vi "experiment control.vi"() -> ()   [LabVIEW 2012] (continued)
                  tunnel: w3124 -> [w3135]
                  stop <- w3140 stop-if-true
                  n1342 = Multiply(x=w3136, y=0.001) -> (x*y=w3144:dbl)
                  n1343 = call-poly <vilib>:"DAQmx Create Virtual Channel.vi"("maximum value"=10.0, "minimum value"=0.0, "physical channels"=w3146, "error in"=w3135) -> ("task out"=w3155:refnum<k21>, "error out"=w3154:errorcluster)  [unwired: 10 in]
                  n1344 = Add(x=w3139, y=w3144) -> (x+y=w3143:dbl)
                  n1345 = Max & Min(x=w3139, y=w3134) -> (max(x,y)=w3142:dbl, min(x,y)=w3141:dbl)
                  n1346 = In Range and Coerce(upper limit=w3142, x=w3143, lower limit=w3141) -> (coerced(x)=w3137:dbl)  [unwired: 1 out]
                  n1347 = call-poly <vilib>:"DAQmx Write.vi"("task/channels in"=w3155, "data"=w3137, "error in"=w3154) -> ("task out"=w3151:refnum<k21>, "error out"=w3156:errorcluster)  [unwired: 10 in, 1 out]
                  n1348 = Equal?(x=w3137, y=w3134) -> (x = y?=w3140:bool)
                  n1349 = call <vilib>:"DAQmx Start Task.vi"("task/channels in"=w3151, "error in"=w3156) -> ("task out"=w3150:refnum<k21>, "error out"=w3149:errorcluster)  [unwired: 12 in]
                  n1350 = call <vilib>:"DAQmx Clear Task.vi"("task in"=w3150, "error in"=w3149) -> ("error out"=w3148:errorcluster)  [unwired: 13 in]
                  n1351 = call "wait.vi"("error in (no error)"=w3148, "ms to wait"=u32 5) -> ("error out (no error)"=w3147:errorcluster)  [unwired: 7 in]
                }
              }
              frame "Stella" {
                n1352 = disable-structure shown="Disabled" {
                  disable-tunnel: w3158 -> [w3160 w3190]
                  disable-tunnel: [w3159 w3190] -> w3157
                  frame Disabled {
                    n1353 = flat-sequence {
                      tunnel: [w3165] -> w3162
                      tunnel: [w3164] -> w3161
                      tunnel: w3160 -> [w3163]
                      tunnel: w3162 -> [w3172]
                      tunnel: w3161 -> [w3170]
                      tunnel: [w3169] -> w3159
                      frame #0 {
                        n1354 = local read "Stella"() -> (w3168:T20)
                        n1355 = Unbundle By Name(w3168) -> ("scan start"=w3166:dbl)
                        n1356 = Bundle By Name(cluster=w3168, "setpoint"=w3166, "progress"=u8 0 ("number")) -> (w3165:T20)
                        n1357 = shared-variable "My Computer\\shared variables.lvlib\\lisa setpoint"(w3166, error in=w3163) -> (error out=w3164:errorcluster)
                        n1358 = local write "Stella"(w3165) -> ()
                      }
                      frame #1 {
                        n1359 = Tick Count (ms)() -> (millisecond timer value=w3171:u32)
                        n1360 = while {
                          tunnel: w3172 -> [w3189]
                          tunnel: w3171 -> [w3184]
                          shift-right: [w3173] -> w3169
                          shift-left: w3170 -> [w3174]
                          stop <- w3179 stop-if-true
                          n1361 = shared-variable "My Computer\\shared variables.lvlib\\lisa wavelength"(error in=w3174) -> (w3175:dbl, error out=w3173:errorcluster)
                          n1362 = Unbundle By Name(w3189) -> ("setpoint"=w3178:dbl, "lock tolerance"=w3186:dbl)
                          n1363 = Subtract(x=w3175, y=w3178) -> (x-y=w3188:dbl)
                          n1364 = Absolute Value(x=w3188) -> (abs(x)=w3187:dbl)
                          n1365 = Less?(x=w3187, y=w3186) -> (x < y?=w3180:bool)
                          n1366 = local read "Stella"() -> (w3176:T20)
                          n1367 = Bundle By Name(cluster=w3176, "wavelength"=w3175) -> (w3177:T20)
                          n1368 = Tick Count (ms)() -> (millisecond timer value=w3185:u32)
                          n1369 = Subtract(x=w3185, y=w3184) -> (x-y=w3183:u32)
                          n1370 = Greater?(x=w3183, y=u32 10000) -> (0:w3181:bool)
                          n1371 = local write "Stella"(w3177) -> ()
                          n1372 = Or(x=w3180, y=w3181) -> (x .or. y?=w3179:bool)
                        }
                      }
                    }
                  }
                  frame Enabled {
                  }
                }
              }
              frame "Jessica" {
                n1373 = disable-structure shown="Enabled" {
                  disable-tunnel: w3192 -> [w3194 w3224]
                  disable-tunnel: [w3193 w3224] -> w3191
                  frame Disabled {
                    n1374 = flat-sequence {
                      tunnel: [w3199] -> w3196
                      tunnel: [w3198] -> w3195
                      tunnel: w3194 -> [w3197]
                      tunnel: w3196 -> [w3206]
                      tunnel: w3195 -> [w3204]
                      tunnel: [w3203] -> w3193
                      frame #0 {
                        n1375 = local read "Jessica"() -> (w3202:T17)
                        n1376 = Unbundle By Name(w3202) -> ("scan start"=w3200:dbl)
                        n1377 = Bundle By Name(cluster=w3202, "setpoint"=w3200, "progress"=u8 0 ("number")) -> (w3199:T17)
                        n1378 = shared-variable "My Computer\\shared variables.lvlib\\jessica setpoint"(w3200, error in=w3197) -> (error out=w3198:errorcluster)
                        n1379 = local write "Jessica"(w3199) -> ()
                      }
                      frame #1 {
                        n1380 = Tick Count (ms)() -> (millisecond timer value=w3205:u32)
                        n1381 = while {
                          tunnel: w3206 -> [w3223]
                          tunnel: w3205 -> [w3218]
                          shift-right: [w3207] -> w3203
                          shift-left: w3204 -> [w3208]
                          stop <- w3213 stop-if-true
                          n1382 = shared-variable "My Computer\\shared variables.lvlib\\jessica wavelength"(error in=w3208) -> (w3209:dbl, error out=w3207:errorcluster)
                          n1383 = Unbundle By Name(w3223) -> ("setpoint"=w3212:dbl, "lock tolerance"=w3220:dbl)
                          n1384 = Subtract(x=w3209, y=w3212) -> (x-y=w3222:dbl)
                          n1385 = Absolute Value(x=w3222) -> (abs(x)=w3221:dbl)
                          n1386 = Less?(x=w3221, y=w3220) -> (x < y?=w3214:bool)
                          n1387 = local read "Jessica"() -> (w3210:T17)
                          n1388 = Bundle By Name(cluster=w3210, "wavelength"=w3209) -> (w3211:T17)
                          n1389 = Tick Count (ms)() -> (millisecond timer value=w3219:u32)
                          n1390 = Subtract(x=w3219, y=w3218) -> (x-y=w3217:u32)
                          n1391 = Greater?(x=w3217, y=u32 10000) -> (0:w3215:bool)
                          n1392 = local write "Jessica"(w3211) -> ()
                          n1393 = Or(x=w3214, y=w3215) -> (x .or. y?=w3213:bool)
                        }
                      }
                    }
                  }
                  frame Enabled {
                  }
                }
              }
              frame "Bertha" {
                n1394 = local read "Bertha"() -> (w3229:T22)
                n1395 = Unbundle By Name(w3229) -> ("scan start"=w3227:dbl)
                n1396 = Bundle By Name(cluster=w3229, "setpoint"=w3227, "progress"=u8 0 ("number")) -> (w3228:T22)
                n1397 = local write "Bertha"(w3228) -> ()
              }
              frame "Cora" {
                n1398 = local read "Cora"() -> (w3234:T21)
                n1399 = Unbundle By Name(w3234) -> ("scan start"=w3232:dbl)
                n1400 = Bundle By Name(cluster=w3234, "setpoint"=w3232, "progress"=u8 0 ("number")) -> (w3233:T21)
                n1401 = local write "Cora"(w3233) -> ()
              }
            }
          }
          frame "Laser: Read Wavelength" {
            n1402 = case shown="\"Stella\"" w3238 {
              tunnel: [w3240 w3242 w3270 w3289 w3308 w3337] -> w3236
              tunnel: w3237 -> [w3240 w3241 w3272 w3293 w3307 w3338]
              frame Default {
              }
              frame "Jessica" {
                n1403 = disable-structure shown="Enabled" {
                  disable-tunnel: [w3249 w3264] -> w3242
                  disable-tunnel: w3241 -> [w3253 w3264]
                  frame Enabled {
                    n1404 = disable-structure shown="Enabled" {
                      disable-tunnel: w3253 -> [w3258 w3261]
                      disable-tunnel: [w3257 w3259] -> w3250
                      disable-tunnel: [w3256 w3260] -> w3249
                      frame Disabled {
                        n1405 = shared-variable "My Computer\\shared variables.lvlib\\luna_wavelength"(error in=w3258) -> (w3257:dbl, error out=w3256:errorcluster)
                      }
                      frame Enabled {
                        n1406 = call "read_cw.vi"("error in"=w3261, "cw_laser"="cw3") -> ("error out"=w3260:errorcluster, "slot"=w3262:T101)  [unwired: 8 in]
                        n1407 = Unbundle By Name(w3262) -> ("wavelength"=w3259:dbl)
                      }
                    }
                    n1408 = local read "Jessica"() -> (w3254:T17)
                    n1409 = Unbundle By Name(w3254) -> ("wavelength"=w3251:dbl, "setpoint"=w3245:dbl, "lock tolerance"=w3243:dbl)
                    n1410 = Less Or Equal To 0?(x=w3250) -> (x <= 0?=w3252:bool)
                    n1411 = Select(t=w3251, s=w3252, f=w3250) -> (s? t:f=w3244:dbl)
                    n1412 = Subtract(x=w3245, y=w3244) -> (x-y=w3248:dbl)
                    n1413 = Absolute Value(x=w3248) -> (abs(x)=w3247:dbl)
                    n1414 = Less?(x=w3247, y=w3243) -> (x < y?=w3246:bool)
                    n1415 = Bundle By Name(cluster=w3254, "locked"=w3246, "wavelength"=w3244) -> (w3255:T17)
                    n1416 = local write "Jessica"(w3255) -> ()
                  }
                  frame Disabled {
                  }
                }
              }
              frame "Toptica" {
                n1417 = local read "Toptica"() -> (w3276:T19)
                n1418 = disable-structure shown="Enabled" {
                  disable-tunnel: [w3280 w3281] -> w3273
                  disable-tunnel: w3272 -> [w3279 w3284]
                  disable-tunnel: [w3278 w3283] -> w3266
                  frame Disabled {
                    n1419 = shared-variable "My Computer\\shared variables.lvlib\\toptica_wavelength"(error in=w3279) -> (w3280:dbl, error out=w3278:errorcluster)
                  }
                  frame Enabled {
                    n1420 = call "read_cw.vi"("error in"=w3284, "cw_laser"="cw1") -> ("error out"=w3283:errorcluster, "slot"=w3282:T101)  [unwired: 8 in]
                    n1421 = Unbundle By Name(w3282) -> ("wavelength"=w3281:dbl)
                  }
                }
                n1422 = Unbundle By Name(w3276) -> ("wavelength"=w3274:dbl)
                n1423 = Less Or Equal To 0?(x=w3273) -> (x <= 0?=w3275:bool)
                n1424 = Select(t=w3274, s=w3275, f=w3273) -> (s? t:f=w3271:dbl)
                n1425 = local read "toptica:task:skip"() -> (w3265:refnum<k21>)
                n1426 = call-poly <vilib>:"DAQmx Read.vi"("task/channels in"=w3265, "error in"=w3266) -> ("data"=w3268:dbl, "error out"=w3270:errorcluster)  [unwired: 11 in, 1 out]
                n1427 = Less?(x=w3268, y=1.8) -> (x < y?=w3269:bool)
                n1428 = Bundle By Name(cluster=w3276, "locked"=w3269, "wavelength"=w3271) -> (w3277:T19)
                n1429 = local write "Toptica"(w3277) -> ()
              }
              frame "Stella" {
                n1430 = disable-structure shown="Enabled" {
                  disable-tunnel: [w3301 w3303] -> w3294
                  disable-tunnel: w3293 -> [w3300 w3302]
                  disable-tunnel: [w3299 w3304] -> w3287
                  frame Disabled {
                    n1431 = shared-variable "My Computer\\shared variables.lvlib\\stella_wavelength"(error in=w3300) -> (w3301:dbl, error out=w3299:errorcluster)
                  }
                  frame Enabled {
                    n1432 = call "read_cw.vi"("error in"=w3302, "cw_laser"="cw0") -> ("error out"=w3304:errorcluster, "slot"=w3305:T101)  [unwired: 8 in]
                    n1433 = Unbundle By Name(w3305) -> ("wavelength"=w3303:dbl)
                  }
                }
                n1434 = local read "Stella"() -> (w3297:T20)
                n1435 = Unbundle By Name(w3297) -> ("wavelength"=w3295:dbl)
                n1436 = Less Or Equal To 0?(x=w3294) -> (x <= 0?=w3296:bool)
                n1437 = Select(t=w3295, s=w3296, f=w3294) -> (s? t:f=w3292:dbl)
                n1438 = local read "stella:task:skip"() -> (w3286:refnum<k21>)
                n1439 = call-poly <vilib>:"DAQmx Read.vi"("task/channels in"=w3286, "error in"=w3287) -> ("data"=w3291:dbl, "error out"=w3289:errorcluster)  [unwired: 11 in, 1 out]
                n1440 = Less?(x=w3291, y=1.8) -> (x < y?=w3288:bool)
                n1441 = Bundle By Name(cluster=w3297, "locked"=w3288, "wavelength"=w3292) -> (w3298:T20)
                n1442 = local write "Stella"(w3298) -> ()
              }
              frame "Cora" {
                n1443 = disable-structure shown="Enabled" {
                  disable-tunnel: [w3309 w3330] -> w3308
                  disable-tunnel: w3307 -> [w3312 w3330]
                  frame Enabled {
                    n1444 = disable-structure shown="Enabled" {
                      disable-tunnel: [w3319 w3320] -> w3313
                      disable-tunnel: w3312 -> [w3318 w3323]
                      disable-tunnel: [w3317 w3322] -> w3309
                      frame Disabled {
                        n1445 = shared-variable "My Computer\\shared variables.lvlib\\cora_wavelength"(error in=w3318) -> (w3319:dbl, error out=w3317:errorcluster)
                      }
                      frame Enabled {
                        n1446 = disable-structure shown="Enabled" {
                          disable-tunnel: "pulse1" ("cw_laser") -> [w3328 _]
                          disable-tunnel: w3323 -> [w3327 w3329]
                          disable-tunnel: [w3326 w3329] -> w3322
                          disable-tunnel: [w3325 _] -> w3321
                          frame Disabled {
                            n1447 = call "read_pulsed.vi"("error in"=w3327, "pulsed_laser"=w3328) -> ("error out"=w3326:errorcluster, "slot"=w3325:T102)  [unwired: 8 in]
                          }
                          frame Enabled {
                          }
                        }
                        n1448 = Unbundle By Name(w3321) -> ("wavelength"=w3320:dbl)
                      }
                    }
                    n1449 = local read "Cora"() -> (w3315:T21)
                    n1450 = Unbundle By Name(w3315) -> ("wavelength"=w3310:dbl)
                    n1451 = Less Or Equal To 0?(x=w3313) -> (x <= 0?=w3314:bool)
                    n1452 = Select(t=w3310, s=w3314, f=w3313) -> (s? t:f=w3311:dbl)
                    n1453 = Bundle By Name(cluster=w3315, "wavelength"=w3311) -> (w3316:T21)
                    n1454 = local write "Cora"(w3316) -> ()
                  }
                  frame Disabled {
                  }
                }
              }
              frame "Bertha" {
                n1455 = local read "Bertha"() -> (w3334:T22)
                n1456 = Unbundle By Name(w3334) -> ("wavelength"=w3333:dbl)
                n1457 = disable-structure shown="Enabled" {
                  disable-tunnel: [w3341 w3342] -> w3331
                  disable-tunnel: w3338 -> [w3340 w3345]
                  disable-tunnel: [w3339 w3344] -> w3337
                  frame Disabled {
                    n1458 = shared-variable "My Computer\\shared variables.lvlib\\cora_wavelength"(error in=w3340) -> (w3341:dbl, error out=w3339:errorcluster)
                  }
                  frame Enabled {
                    n1459 = disable-structure shown="Disabled" {
                      disable-tunnel: "pulse1" ("cw_laser") -> [w3350 _]
                      disable-tunnel: w3345 -> [w3349 w3351]
                      disable-tunnel: [w3348 w3351] -> w3344
                      disable-tunnel: [w3347 _] -> w3343
                      frame Disabled {
                        n1460 = call "read_pulsed.vi"("error in"=w3349, "pulsed_laser"=w3350) -> ("error out"=w3348:errorcluster, "slot"=w3347:T102)  [unwired: 8 in]
                      }
                      frame Enabled {
                      }
                    }
                    n1461 = Unbundle By Name(w3343) -> ("wavelength"=w3342:dbl)
                  }
                }
                n1462 = Less Or Equal To 0?(x=w3331) -> (x <= 0?=w3336:bool)
                n1463 = Select(t=w3333, s=w3336, f=w3331) -> (s? t:f=w3332:dbl)
                n1464 = Bundle By Name(cluster=w3334, "wavelength"=w3332) -> (w3335:T22)
                n1465 = local write "Bertha"(w3335) -> ()
              }
            }
          }
          frame "Laser: Initialize DAC" {
            n1466 = local read "Toptica"() -> (w3359:T19)
            n1467 = local read "Stella"() -> (w3358:T20)
            n1468 = Unbundle By Name(w3359) -> ("AI Channel"=w3360:tag)
            n1469 = Unbundle By Name(w3358) -> ("AI Channel"=w3357:tag)
            n1470 = call-poly <vilib>:"DAQmx Create Virtual Channel.vi"("physical channels"=w3360, "error in"=w3354) -> ("task out"=→"toptica:task:skip":refnum<k21>, "error out"=w3356:errorcluster)  [unwired: 12 in]
            n1471 = call-poly <vilib>:"DAQmx Create Virtual Channel.vi"("physical channels"=w3357, "error in"=w3356) -> ("task out"=→"stella:task:skip":refnum<k21>, "error out"=w3355:errorcluster)  [unwired: 12 in]
          }
          frame "Laser: Close DAC" {
            n1472 = local read "toptica:task:skip"() -> (w3363:refnum<k21>)
            n1473 = local read "stella:task:skip"() -> (w3364:refnum<k21>)
            n1474 = call <vilib>:"DAQmx Clear Task.vi"("task in"=w3363, "error in"=w3365) -> ("error out"=w3367:errorcluster)  [unwired: 13 in]
            n1475 = call <vilib>:"DAQmx Clear Task.vi"("task in"=w3364, "error in"=w3367) -> ("error out"=w3366:errorcluster)  [unwired: 13 in]
          }
          frame "---------- Debug ----------" {
            # "Template Separator\n(You can make a copy of, or modify, this frame)"
          }
          frame "Debug: Popup" {
            # "Prints the argument to a popup dialog box. Careful! If you get stuck in a loop this can hang the program."
            n1476 = One Button Dialog(message=w3375) -> (true=w3374:bool)  [unwired: 1 in]
            n1477 = flat-sequence {
              tunnel: w3374 -> [_]
              frame #0 {
                # "This delay is added in to make it difficult for the user to create and infinite chain of popups"
                n1478 = Wait (ms)(milliseconds to wait=u32 200) -> ()  [unwired: 1 out]
              }
            }
          }
          frame "Debug: Console" {
            # "Prints the argument to the console."
            n1479 = flat-sequence {
              tunnel: w3380 -> [w3383]
              frame #0 {
                n1480 = local read "stdout"() -> (w3385:string)
                n1481 = Concatenate Strings(w3385, "\r\n", w3383) -> (w3386:string)
                n1482 = local write "stdout"(w3386) -> ()
              }
              frame #1 {
                n1483 = property on="stdout" class="Str"("Text.Scroll Position"=u32 4294967295) -> ()  [unwired: 2 in, 2 out]
              }
            }
          }
          frame "---------- Wavemaster ----------" {
            # "Template Separator\n(You can make a copy of, or modify, this frame)"
          }
          frame "Wavemeter: Initialise" {
            n1484 = local read "Wavemaster"() -> (w3397:T23)
            n1485 = Unbundle By Name(w3397) -> ("Serial Port"=w3399:refnum<visa-resource-name>)
            n1486 = Bundle By Name(cluster=T46 {"VISA resource name"="COM6", "baud rate"=9600, "data bits"=8, "parity"=0, "stop bits"=10, "flow control"=2, "termination char\n(0xA = '\\n' = LF)"=10, "timeout (ms)"=1000, "End write with termination character?"=TRUE, "End read on termination character?"=TRUE} ("Serial Settings"), "VISA resource name"=w3399) -> (w3398:T46)
            n1487 = call "Wmeter Initialize.vi"("error in"=w3402, "Serial Settings"=w3398) -> ("error out (no error)"=w3401:errorcluster, "VISA RName out"=w3396:refnum<visa-resource-name>)  [unwired: 8 in]
            n1488 = Unbundle By Name(w3401) -> ("status"=w3394:bool)
            n1489 = Not(x=w3394) -> (.not. x?=w3393:bool)
            n1490 = Bundle By Name(cluster=w3397, "VISA Name"=w3396, "Detected"=w3393) -> (w3395:T23)
            n1491 = local write "Wavemaster"(w3395) -> ()
            n1492 = Enqueue Element(queue=w3392, element="Debug: Console >> Initializing Wavemeter" ("State(s) at Back (\"\")")) -> ()  [unwired: 2 in, 3 out]
          }
          frame "Wavemeter: Start" {
            n1493 = local read "Wavemaster"() -> (w3408:T23)
            n1494 = Unbundle By Name(w3408) -> ("VISA Name"=w3407:refnum<visa-resource-name>, "Detected"=w3406:bool)
            n1495 = case shown="True" w3406 {
              tunnel: [w3413 w3420] -> w3409
              tunnel: w3410 -> [w3413 w3419]
              tunnel: w3408 -> [_ w3418]
              tunnel: w3407 -> [_ w3415]
              tunnel: ["Debug: Console >> Can't Find Wavemeter" ("State(s) at Back (\"\")") "Debug: Console >> Starting Wavemeter" ("State(s) at Back (\"\")")] -> w3405
              frame False {
              }
              frame True {
                n1496 = call "Wmeter Start.vi"("error in"=w3419, "WMeter"=w3415) -> ("error out"=w3420:errorcluster, "WMeter out"=w3417:refnum<visa-resource-name>)  [unwired: 8 in]
                n1497 = Bundle By Name(cluster=w3418, "VISA Name"=w3417) -> (w3416:T23)
                n1498 = local write "Wavemaster"(w3416) -> ()
              }
            }
            n1499 = Enqueue Element At Opposite End(queue=w3404, element=w3405) -> ()  [unwired: 2 in, 3 out]
          }
          frame "Wavemeter: Set Units" {
            n1500 = local read "Wavemaster"() -> (w3426:T23)
            n1501 = Unbundle By Name(w3426) -> ("VISA Name"=w3425:refnum<visa-resource-name>, "Units"=w3424:string, "Detected"=w3423:bool)
            n1502 = case shown="True" w3423 {
              tunnel: [w3430 w3439] -> w3427
              tunnel: w3428 -> [w3430 w3438]
              tunnel: w3426 -> [_ w3437]
              tunnel: w3425 -> [_ w3434]
              tunnel: [_ w3432] -> w3421
              tunnel: w3424 -> [_ w3431]
              frame False {
              }
              frame True {
                n1503 = call "Wmeter Units.vi"("error in"=w3438, "Combo Box"=w3431, "WMeter"=w3434) -> ("error out"=w3439:errorcluster, "WMeter out"=w3436:refnum<visa-resource-name>)  [unwired: 7 in]
                n1504 = Bundle By Name(cluster=w3437, "VISA Name"=w3436) -> (w3435:T23)
                n1505 = local write "Wavemaster"(w3435) -> ()
                n1506 = Concatenate Strings("Debug: Console >> Changing Wavemeter units to " ("State(s) at Back (\"\")"), w3431) -> (w3432:string)
              }
            }
            n1507 = Enqueue Element At Opposite End(queue=w3422, element=w3421) -> ()  [unwired: 2 in, 3 out]
          }
          frame "Wavemeter: Read" {
            n1508 = local read "Wavemaster"() -> (w3444:T23)
            n1509 = Unbundle By Name(w3444) -> ("VISA Name"=w3443:refnum<visa-resource-name>, "Wavelength"=w3442:dbl, "Detected"=w3441:bool)
            n1510 = case shown="True" w3441 {
              tunnel: [w3448 w3458] -> w3445
              tunnel: w3446 -> [w3448 w3457]
              tunnel: w3444 -> [_ w3456]
              tunnel: w3443 -> [_ w3453]
              tunnel: w3442 -> [_ w3450]
              frame False {
              }
              frame True {
                n1511 = call "Wmeter Read.vi"("error in"=w3457, "WMeter"=w3453) -> ("error out"=w3458:errorcluster, "Wavelength"=w3451:dbl, "WMeter out"=w3455:refnum<visa-resource-name>)  [unwired: 7 in]
                n1512 = Greater Than 0?(x=w3451) -> (x > 0?=w3449:bool)
                n1513 = Select(t=w3451, s=w3449, f=w3450) -> (s? t:f=w3452:dbl)
                n1514 = Bundle By Name(cluster=w3456, "VISA Name"=w3455, "Wavelength"=w3452, "Reading"=w3449) -> (w3454:T23)
                n1515 = local write "Wavemaster"(w3454) -> ()
              }
            }
          }
          frame "Wavemeter: Stop" {
            n1516 = local read "Wavemaster"() -> (w3463:T23)
            n1517 = Unbundle By Name(w3463) -> ("VISA Name"=w3462:refnum<visa-resource-name>, "Detected"=w3461:bool)
            n1518 = case shown="True" w3461 {
              tunnel: [w3467 w3474] -> w3464
              tunnel: w3465 -> [w3467 w3473]
              tunnel: w3463 -> [_ w3472]
              tunnel: w3462 -> [_ w3469]
              tunnel: [_ "Debug: Console >> Stopping Wavemeter" ("State(s) at Back (\"\")")] -> w3460
              frame False {
              }
              frame True {
                n1519 = call "Wmeter Stop.vi"("error in"=w3473, "WMeter"=w3469) -> ("error out"=w3474:errorcluster, "WMeter out"=w3471:refnum<visa-resource-name>)  [unwired: 8 in]
                n1520 = Bundle By Name(cluster=w3472, "VISA Name"=w3471) -> (w3470:T23)
                n1521 = local write "Wavemaster"(w3470) -> ()
              }
            }
            n1522 = Enqueue Element At Opposite End(queue=w3459, element=w3460) -> ()  [unwired: 2 in, 3 out]
          }
          frame "Wavemeter: Close" {
            n1523 = local read "Wavemaster"() -> (w3479:T23)
            n1524 = Unbundle By Name(w3479) -> ("VISA Name"=w3478:refnum<visa-resource-name>, "Detected"=w3477:bool)
            n1525 = case shown="True" w3477 {
              tunnel: [w3483 w3487] -> w3480
              tunnel: w3481 -> [w3483 w3486]
              tunnel: w3478 -> [_ w3485]
              tunnel: [_ "Debug: Console >> Closing Wavemeter Resource" ("State(s) at Back (\"\")")] -> w3475
              frame False {
              }
              frame True {
                n1526 = call "Wmeter Close.vi"("error in"=w3486, "WMeter"=w3485) -> ("error out"=w3487:errorcluster)  [unwired: 9 in]
              }
            }
            n1527 = Enqueue Element(queue=w3476, element=w3475) -> ()  [unwired: 2 in, 3 out]
          }
          frame "---------- DIO64 ----------" {
            # "Template Separator\n(You can make a copy of, or modify, this frame)"
          }
          frame "DIO64: Initialise" {
            # "Initialize DIO64 Board"
            n1528 = case shown="\"Windows x64\"" T47."Windows x64" ("App.TargetOS") {
              tunnel: [w3501 w3508 w3516] -> w3495
              tunnel: w3497 -> [w3500 w3509 w3517]
              tunnel: "VISA resource name" -> [w3499 _ _]
              frame "Windows x64" {
                n1529 = call "DIO64 OpenResource.vi"("board in"=u16 0, "resourceName"=w3499, "error in (no error)"=w3500) -> ("board out"=w3502:u16, "error out"=w3504:errorcluster)  [unwired: 11 in]
                n1530 = call "DIO64 Load.vi"("board in"=w3502, "input hint"=0, "output hint"=4, "filename"=path "C:/DIO64/DIO64.CAT", "error in (no error)"=w3504) -> ("error out"=w3501:errorcluster)  [unwired: 9 in, 1 out]
              }
              frame "Windows 95/NT" {
                n1531 = call "DIO64 Open.vi"("board in"=u16 0, "error in (no error)"=w3509) -> ("board out"=w3510:u16, "error out"=w3512:errorcluster)  [unwired: 12 in]
                n1532 = call "DIO64 Load.vi"("board in"=w3510, "input hint"=0, "output hint"=4, "error in (no error)"=w3512) -> ("error out"=w3508:errorcluster)  [unwired: 10 in, 1 out]
              }
              frame "invalid OS target", Default {
                n1533 = Merge Errors(errorcluster {"status"=TRUE, "code"=0, "source"="DIO64: Unknown OS!!"} ("error constant"), w3517) -> (w3516:errorcluster)
              }
            }
            n1534 = case shown="No Error" w3495 {
              tunnel: w3495 -> [w3518 w3522]
              tunnel: [w3518 w3519] -> w3496
              frame No Error {
              }
              frame Error {
                n1535 = call <vilib>:"Error Cluster From Error Code.vi"("error in (no error)"=w3522, "error message (\"\")"="DIO64 Not Found!" ("error message (\"\")"), "error code (0)"=0) -> ("error out"=w3519:errorcluster)  [unwired: 6 in]
              }
            }
            n1536 = Enqueue Element(queue=w3491, element="Debug: Console >> Initializing DIO64") -> ()  [unwired: 2 in, 3 out]
          }
          frame "DIO64: Prepare" {
            n1537 = case shown="\"0\", \"1\", \"10\", \"11\", \"12\", \"2\", \"3\", \"4\", \"5\", \"6\", \"7\", \"8\", \"9\", Default" w3526 {
              tunnel: w3526 -> [w3536 _]
              tunnel: [w3535 w3538] -> w3524
              tunnel: w3525 -> [w3534 w3538]
              frame "0", "1", "10", "11", "12", "2", "3", "4", "5", "6", "7", "8", "9", Default {
                n1538 = Decimal String To Number(string=w3536) -> (number=w3531:i32)  [unwired: 2 in, 1 out]
                n1539 = local read "Frames and Rep Rate"() -> (w3537:cluster{"Frames":i32, "Repetition Rate":dbl})
                n1540 = local read "DIO64 Tasks"() -> (w3532:T4)
                n1541 = local read "DIO64"() -> (w3533:T3)
                n1542 = Unbundle By Name(w3537) -> ("Repetition Rate"=w3530:dbl)
                n1543 = call "Parse DIO64v4.vi"("error in"=w3534, "DIO64"=w3533) -> ("error out"=w3535:errorcluster, "times"=w3529:T37)  [unwired: 7 in]
                n1544 = call "Prepare DIO64v4.vi"("Repetition Rate"=w3530, "chop"=w3531, "times"=w3529, "DIO64 Tasks"=w3532) -> ("DIO64 Debug"=w3528:T36)  [unwired: 6 in]
                n1545 = local write "dio64:debug2"(w3528) -> ()
                n1546 = local write "dio64:debug1"(w3529) -> ()
              }
              frame "True" {
              }
            }
          }
          frame "DIO64: Update Graph" {
            n1547 = local read "Frames and Rep Rate"() -> (w3569:cluster{"Frames":i32, "Repetition Rate":dbl})
            n1548 = local read "DIO64 Tasks"() -> (w3567:T4)
            n1549 = local read "DIO64"() -> (w3568:T3)
            n1550 = Unbundle By Name(w3569) -> ("Repetition Rate"=w3566:dbl)
            n1551 = call "Parse DIO64v4.vi"("error in"=w3572, "DIO64"=w3568) -> ("error out"=w3571:errorcluster, "times"=w3565:T37)  [unwired: 7 in]
            n1552 = call "Prepare DIO64v4.vi"("Repetition Rate"=w3566, "chop"="Column", "times"=w3565, "DIO64 Tasks"=w3567) -> ("DIO64 Debug"=w3551:T36)  [unwired: 6 in]
            n1553 = for {
              tunnel: w3551 -> [w3632] mode=indexing
              tunnel: [w3631] -> w3552 mode=indexing
              tunnel: [w3630] -> w3557 mode=indexing
              tunnel: [w3629] -> w3559 mode=indexing
              tunnel: [w3628] -> w3561 mode=indexing
              tunnel: [w3627] -> w3563 mode=indexing
              n1554 = Unbundle By Name(w3632) -> ("Begin (ms)"=w3631:dbl, "DIO64 Line 1"=w3630:bool[], "DIO64 Line 2"=w3629:bool[], "DIO64 Line 3"=w3628:bool[], "DIO64 Line 4"=w3627:bool[])
            }
            n1555 = Transpose 2D Array(2D array=w3557) -> (transposed array=w3558:bool[][])
            n1556 = Transpose 2D Array(2D array=w3559) -> (transposed array=w3560:bool[][])
            n1557 = Transpose 2D Array(2D array=w3561) -> (transposed array=w3562:bool[][])
            n1558 = Transpose 2D Array(2D array=w3563) -> (transposed array=w3564:bool[][])
            n1559 = for {
              tunnel: w3558 -> [w3624] mode=indexing
              tunnel: w3552 -> [w3613]
              tunnel: [w3626] -> w3553 mode=indexing
              tunnel: w3560 -> [w3621] mode=indexing
              tunnel: w3562 -> [w3619] mode=indexing
              tunnel: w3564 -> [w3617] mode=indexing
              tunnel: [w3612] -> w3554 mode=indexing
              tunnel: [w3611] -> w3555 mode=indexing
              tunnel: [w3610] -> w3556 mode=indexing
              n1560 = Boolean To (0,1)(Boolean=w3624) -> (0, 1=w3623:i16[])
              n1561 = Boolean To (0,1)(Boolean=w3621) -> (0, 1=w3622:i16[])
              n1562 = Boolean To (0,1)(Boolean=w3619) -> (0, 1=w3620:i16[])
              n1563 = Boolean To (0,1)(Boolean=w3617) -> (0, 1=w3618:i16[])
              n1564 = To Double Precision Float(number=w3623) -> (double precision float=w3625:dbl[])
              n1565 = To Double Precision Float(number=w3622) -> (double precision float=w3614:dbl[])
              n1566 = To Double Precision Float(number=w3620) -> (double precision float=w3615:dbl[])
              n1567 = To Double Precision Float(number=w3618) -> (double precision float=w3616:dbl[])
              n1568 = Bundle(w3613, w3625) -> (w3626:cluster{dbl[], dbl[]})  [unwired: 1 in]
              n1569 = Bundle(w3613, w3614) -> (w3612:cluster{dbl[], dbl[]})  [unwired: 1 in]
              n1570 = Bundle(w3613, w3615) -> (w3611:cluster{dbl[], dbl[]})  [unwired: 1 in]
              n1571 = Bundle(w3613, w3616) -> (w3610:cluster{dbl[], dbl[]})  [unwired: 1 in]
            }
            n1572 = local write "dio64:debug1"(w3565) -> ()
            n1573 = local read "Channel Labels"() -> (w3544:T10)
            n1574 = Build Array (concatenate)(w3553, w3554, w3555, w3556) -> (w3547:cluster{dbl[], dbl[]}[])
            n1575 = flat-sequence {
              tunnel: w3542 -> [w3581]
              tunnel: w3541 -> [w3580]
              tunnel: [w3580] -> w3540
              frame #0 {
                "DIO64 Graph" <- w3581
              }
            }
            n1576 = Transpose 2D Array(2D array=w3544) -> (transposed array=w3546:T10)
            n1577 = Reshape Array(w3546, 64 ("dimension size")) -> (w3543:T103)
            n1578 = for {
              tunnel: w3547 -> [w3593] mode=indexing
              tunnel: w3543 -> [w3592] mode=indexing
              shift-right: [w3587] -> _
              shift-left: 0.0 -> [w3588]
              shift-right: [w3582] -> w3542
              shift-left: cluster{dbl[], dbl[]}[] [] -> [w3586]
              shift-right: [w3584] -> w3541
              shift-left: string[] [] -> [w3583]
              n1579 = Unbundle By Name(w3592) -> ("plot"=w3589:bool, "Channel"=w3591:string, "Name"=w3590:string)
              n1580 = Concatenate Strings(w3591, w3590) -> (w3585:string)
              n1581 = case shown="True" w3589 {
                tunnel: w3593 -> [_ w3608]
                tunnel: [w3595 w3603] -> w3582
                tunnel: w3585 -> [_ w3602]
                tunnel: w3588 -> [w3596 w3599]
                tunnel: [w3596 w3598] -> w3587
                tunnel: w3586 -> [w3595 w3605]
                tunnel: [w3594 w3601] -> w3584
                tunnel: w3583 -> [w3594 w3600]
                frame False {
                }
                frame True {
                  n1582 = Unbundle(w3608) -> (w3606:dbl[], w3609:dbl[])
                  n1583 = Add(x=w3609, y=w3599) -> (x+y=w3607:dbl[])
                  n1584 = Bundle(cluster=w3608, w3606, w3607) -> (w3604:cluster{dbl[], dbl[]})
                  n1585 = Subtract(x=w3599, y=1.2) -> (x-y=w3598:dbl)
                  n1586 = Build Array (concatenate)(w3605, w3604) -> (w3603:cluster{dbl[], dbl[]}[])
                  n1587 = Build Array (concatenate)(w3600, w3602) -> (w3601:string[])
                }
              }
            }
            n1588 = for {
              tunnel: w3540 -> [w3575] mode=indexing
              i -> [w3574]
              n1589 = stacked-sequence {
                tunnel: w3575 -> [_ w3577]
                tunnel: w3574 -> [w3576 _]
                frame #0 {
                  n1590 = property on="DIO64 Graph" class="MixedGraph (strict)"("Active Plot"=w3576) -> ()  [unwired: 2 in, 2 out]
                }
                frame #1 {
                  n1591 = property on="DIO64 Graph" class="MixedGraph (strict)"("Plot.Line Width"=u8 3, "Plot.Plot Interpolation"=u8 3, "Plot.Plot Name"=w3577) -> ()  [unwired: 2 in, 2 out]
                }
              }
            }
          }
          frame "DIO64: Run" {
            n1592 = local read "Chops"() -> (w3640:cluster{"Chops":u16[]}[])
            n1593 = Match Pattern(string=w3650, regular expression=",") -> (before substring=w3637:string, after substring=w3636:string)  [unwired: 1 in, 2 out]
            n1594 = Decimal String To Number(string=w3636) -> (number=w3635:i32)  [unwired: 2 in, 1 out]
            n1595 = Index Array(array=w3640, index=w3635) -> (element=w3639:cluster{"Chops":u16[]})
            n1596 = Unbundle By Name(w3639) -> ("Chops"=w3634:u16[])
            n1597 = local read "Frames and Rep Rate"() -> (w3646:cluster{"Frames":i32, "Repetition Rate":dbl})
            n1598 = Equal?(x=w3637, y="Chop") -> (x = y?=w3641:bool)
            n1599 = Array Size(array=w3634) -> (size(s)=w3645:i32)
            n1600 = local write "Current Chops"(w3634) -> ()
            n1601 = Unbundle By Name(w3646) -> ("Frames"=w3648:i32, "Repetition Rate"=w3647:dbl)
            n1602 = Greater Than 0?(x=w3645) -> (x > 0?=w3644:bool)
            n1603 = And(x=w3644, y=w3641) -> (x .and. y?=w3643:bool)
            n1604 = for {
              N: w3648 -> [_]
              tunnel: w3652 -> [w3661]
              tunnel: [w3669] -> w3649 mode=indexing
              tunnel: w3647 -> [w3672]
              tunnel: w3643 -> [w3676]
              tunnel: w3645 -> [w3675]
              tunnel: w3634 -> [w3673]
              tunnel: w3633 -> [w3655]
              i -> [w3674]
              stop <- w3654 stop-if-true
              n1605 = local read "Trap DDS"() -> (w3668:T26)
              n1606 = Get Queue Status(queue=w3655, return elements? (F)=TRUE) -> (elements=w3659:string[])  [unwired: 1 in, 7 out]
              n1607 = Unbundle By Name(w3668) -> ("detected"=w3666:bool)
              n1608 = case shown="True" w3676 {
                tunnel: w3675 -> [_ w3712]
                tunnel: w3674 -> [_ w3711]
                tunnel: w3673 -> [_ w3709]
                tunnel: w3672 -> [_ w3706]
                tunnel: [w3699 w3700] -> w3671
                tunnel: w3661 -> [w3698 w3703]
                tunnel: [w3698 w3702] -> w3660
                frame False {
                  n1609 = local read "dio64:debug2"() -> (w3699:T36)
                }
                frame True {
                  n1610 = Quotient & Remainder(x=w3711, y=w3712) -> (x-y*floor(x/y)=w3710:i32)  [unwired: 1 out]
                  n1611 = Index Array(array=w3709, index=w3710) -> (element=w3707:u16)
                  n1612 = local read "DIO64 Tasks"() -> (w3708:T4)
                  n1613 = local read "DIO64"() -> (w3704:T3)
                  n1614 = call "Parse DIO64v4.vi"("error in"=w3703, "DIO64"=w3704) -> ("error out"=w3702:errorcluster, "times"=w3705:T37)  [unwired: 7 in]
                  n1615 = call "Prepare DIO64v4.vi"("Repetition Rate"=w3706, "chop"=w3707, "times"=w3705, "DIO64 Tasks"=w3708) -> ("DIO64 Debug"=w3700:T36)  [unwired: 6 in]
                  n1616 = case shown="True" "update_debug" {
                    tunnel: w3700 -> [_ w3713]
                    frame False {
                    }
                    frame True {
                      n1617 = local write "dio64:debug2"(w3713) -> ()
                    }
                  }
                }
              }
              n1618 = Search 1D Array(1D array=w3659, element="Abort") -> (index of element=w3657:i32)  [unwired: 1 in]
              n1619 = Greater Or Equal To 0?(x=w3657) -> (x >= 0?=w3654:bool)
              n1620 = Not(x=w3654) -> (.not. x?=w3662:bool)
              n1621 = And(x=w3662, y=w3666) -> (x .and. y?=w3665:bool)
              n1622 = case shown="True" w3665 {
                tunnel: w3668 -> [_ w3697]
                tunnel: w3660 -> [w3678 w3685]
                tunnel: [w3678 w3683] -> w3667
                frame False {
                }
                frame True {
                  w3693 = T104 {"system clock offset"=FALSE, "system clock offset"=FALSE, "open"=FALSE, "open"=FALSE, "multidevice sync mask"=FALSE, "multidevice sync status"=FALSE, "sync master enable"=FALSE, "auto sync enable"=FALSE, "open"=FALSE, "open"=FALSE, "open"=FALSE, "open"=FALSE, "all channel clear phase accumulator"=FALSE, "all channel autoclear phase accumulator"=FALSE, "all channel clear sweep accumulator"=FALSE, "all channel autoclear sweep accumulator"=FALSE} ("Channel Function Register")
                  n1623 = Bundle By Name(cluster=w3693, "all channel clear phase accumulator"=TRUE) -> (w3691:T104)
                  n1624 = Unbundle By Name(w3697) -> ("usb 1"=w3696:refnum<visa-resource-name>, "usb 2"=w3686:refnum<visa-resource-name>)
                  n1625 = call "DDS9959 Set FR2.vi"("error in (no error)"=w3685, "Channel Function Register"=w3691, "VISA resource name"=w3696) -> ("error out"=w3684:errorcluster, "VISA resource name out"=w3690:refnum<visa-resource-name>)  [unwired: 3 in]
                  n1626 = Bundle By Name(cluster=w3693, "all channel clear phase accumulator"=FALSE) -> (w3692:T104)
                  n1627 = call "DDS9959 IO Update.vi"("error in (no error)"=w3684, "VISA resource name"=w3690) -> ("error out"=w3680:errorcluster, "VISA resource name out"=w3689:refnum<visa-resource-name>)  [unwired: 4 in]
                  n1628 = call "DDS9959 Set FR2.vi"("error in (no error)"=w3680, "Channel Function Register"=w3692, "VISA resource name"=w3689) -> ("error out"=w3679:errorcluster)  [unwired: 3 in, 1 out]
                  n1629 = call "DDS9959 Set FR2.vi"("error in (no error)"=w3679, "Channel Function Register"=w3691, "VISA resource name"=w3686) -> ("error out"=w3681:errorcluster, "VISA resource name out"=w3688:refnum<visa-resource-name>)  [unwired: 3 in]
                  n1630 = call "DDS9959 IO Update.vi"("error in (no error)"=w3681, "VISA resource name"=w3688) -> ("error out"=w3682:errorcluster, "VISA resource name out"=w3687:refnum<visa-resource-name>)  [unwired: 4 in]
                  n1631 = call "DDS9959 Set FR2.vi"("error in (no error)"=w3682, "Channel Function Register"=w3692, "VISA resource name"=w3687) -> ("error out"=w3683:errorcluster)  [unwired: 3 in, 1 out]
                }
              }
              n1632 = call "dt_i to 0-t_i.vi"("DIO64 Debug"=w3671) -> ("output cluster"=w3664:cluster{bool[][], bool[][], bool[][], bool[][]}, "DIOArray out 1"=w3670:bool[][], "ti"=w3677:dbl[])  [unwired: 2 in]
              n1633 = call "DIO64 Sequence.vi"("DIO64Addr (0)"=u16 0, "RepRate (Hz)"=w3672, "Time Array (ms)"=w3677, "Set DIO line .."=w3670, "output cluster"=w3664, "error in"=w3667) -> ("error out"=w3669:errorcluster)  [unwired: 9 in]
            }
            n1634 = Merge Errors(w3649) -> (w3651:errorcluster)
          }
          frame "DIO64: Override" {
            w3720 = 10.0 ("Begin (ms)")
            n1635 = local read "DIO64 Override"() -> (w3725:T35)
            n1636 = Unbundle By Name(w3725) -> ("DIO64 Line 1"=w3719:bool[], "DIO64 Line 2"=w3718:bool[], "DIO64 Line 3"=w3717:bool[], "DIO64 Line 4"=w3716:bool[])
            n1637 = Bundle("Begin (ms)"=0.0, "Begin (ms)"=w3720, "DIO64 Line 1"=w3719, "DIO64 Line 2"=w3718, "DIO64 Line 3"=w3717, "DIO64 Line 4"=w3716) -> (w3722:T105)  [unwired: 1 in]
            n1638 = Bundle("Begin (ms)"=w3720, "Begin (ms)"=w3720, "DIO64 Line 1"=w3719, "DIO64 Line 2"=w3718, "DIO64 Line 3"=w3717, "DIO64 Line 4"=w3716) -> (w3723:T105)  [unwired: 1 in]
            n1639 = Build Array(w3722, w3723) -> (w3724:T106)
            n1640 = call "dt_i to 0-t_i.vi"("DIO64 Debug"=w3724) -> ("output cluster"=w3727:cluster{bool[][], bool[][], bool[][], bool[][]}, "DIOArray out 1"=w3728:bool[][], "ti"=w3729:dbl[])  [unwired: 2 in]
            n1641 = call "DIO64 Sequence.vi"("DIO64Addr (0)"=u16 0, "RepRate (Hz)"=10000.0, "Time Array (ms)"=w3729, "Set DIO line .."=w3728, "output cluster"=w3727, "error in"=w3731) -> ("error out"=w3730:errorcluster)  [unwired: 9 in]
          }
          frame "DIO64: Trigger" {
            w3738 = bool[] [FALSE, FALSE, FALSE, FALSE, FALSE, FALSE, FALSE, FALSE, FALSE, FALSE, FALSE, FALSE, FALSE, FALSE, FALSE, FALSE] ("DIO64 Line 4")
            w3747 = 10.0 ("Begin (ms)")
            n1642 = String Subset(string=w3758, length (rest)=1 ("length (rest)")) -> (substring=w3744:string)  [unwired: 1 in]
            n1643 = Decimal String To Number(string=w3758, offset=1 ("offset (0)")) -> (number=w3742:i32)  [unwired: 1 in, 1 out]
            n1644 = In Range and Coerce(upper limit=15, x=w3742, lower limit=0) -> (coerced(x)=w3739:i32)  [unwired: 1 out]
            n1645 = case shown="\"A\", Default" w3744 {
              tunnel: w3739 -> [w3765 w3769 w3773 w3777]
              tunnel: w3738 -> [w3762 w3766 w3770 w3774]
              tunnel: [w3763 w3766 w3770 w3774] -> w3737
              tunnel: [w3762 w3767 w3770 w3774] -> w3736
              tunnel: [w3762 w3766 w3771 w3774] -> w3735
